vi "perform asynchronous fault handling.vi"(0 "module in":T2, 1 "fault fifo":refnum<k33>, 2 "error classification":T1, 3 "iteration":u64, 5 "module ref in":refnum<data-value>, 7 "code":i32, 9 "fault handling in":T4, 11 "run flags in":u8, 12 "engine error in":errorcluster, 13 "engine reference":i32, 14 "cfg ref":refnum<data-value>) -> (4 "module out":T2, 6 "go to safe state":bool, 8 "code out":i32, 10 "engine error out":errorcluster, 15 "run flags out":u8)   [LabVIEW 2013, in "main engine.lvlib"]
uses:
  main engine/main engine.lvlib
  fault handling spec.ctl
  Configuration/Error Actions.ctl
  rt fault.ctl
  <vilib>/NI/Tag Bus Module Framework/runtime/error classification.ctl
  <vilib>/NI/Tag Bus Module Framework/module configuration/TBM module configuration.lvclass
  <vilib>/NI/Tag Bus Module Framework/runtime/TBM module execution interface.lvclass
  async executor/asynchronous executor reference.ctl
  async executor/message to executor.ctl
  async command notification.ctl
  <vilib>/NI/Tag Bus/table/data table.ctl
  async error info.ctl
  <vilib>/NI/Tag Bus/buffer exchange/buffer reference.ctl
  Configuration/Standard Engine Configuration.lvclass
  <vilib>/NI/Tag Bus/table/data table.lvlib
  <vilib>/NI/Tag Bus/buffer exchange/tag bus buffer exchange.lvlib
  async executor/async executor.lvlib
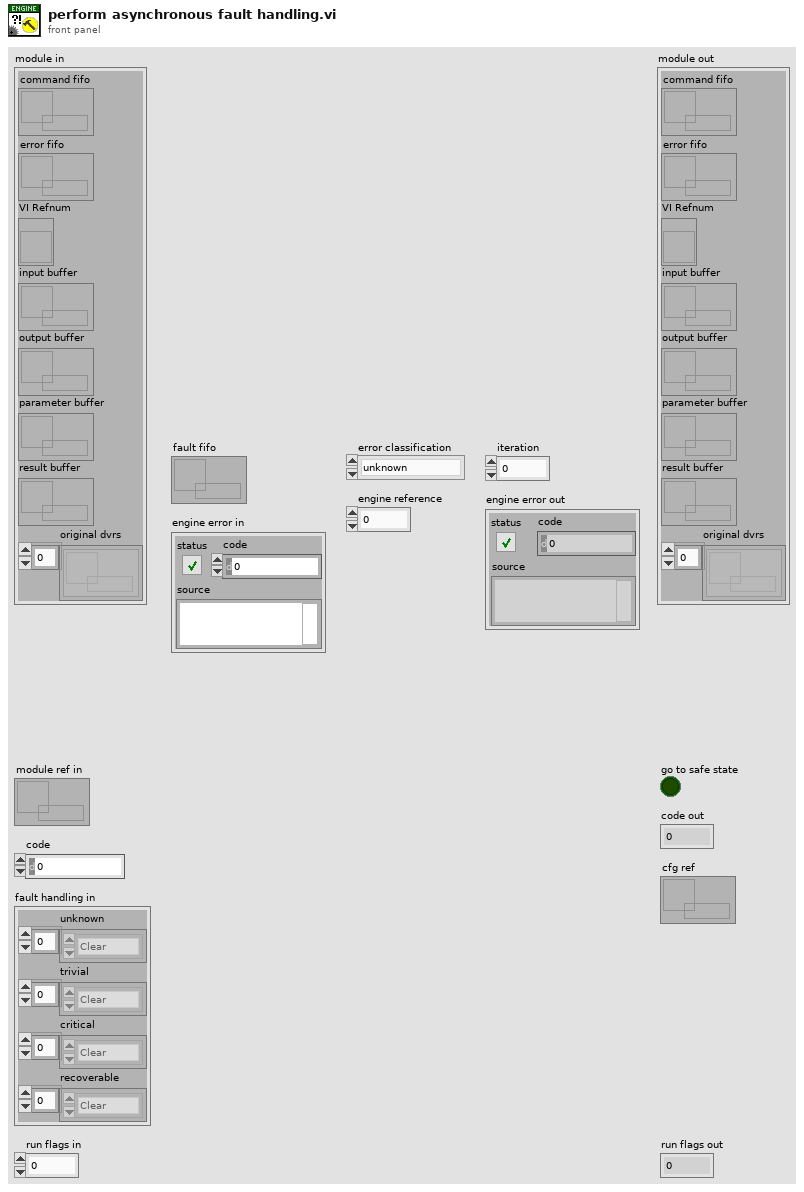
[diagram p1: front panel]
types:
  T1 = typedef "TBM module execution interface.lvclass/error classification.ctl" = enum16{"unknown", "none", "trivial", "recoverable", "critical"}
  T2 = typedef "async executor.lvlib/asynchronous executor reference.ctl" = cluster{"command fifo":refnum<k33>, "error fifo":refnum<k33>, "VI Refnum":refnum<vi>, "input buffer":refnum<k33>, "output buffer":refnum<k33>, "parameter buffer":refnum<k33>, "result buffer":refnum<k33>, "original dvrs":T3[]}
  T3 = typedef "tag bus buffer exchange.lvlib/buffer reference.ctl" = refnum<data-value>
  T4 = typedef "main engine.lvlib/fault handling spec.ctl" = cluster{"unknown":T5[], "trivial":T5[], "critical":T5[], "recoverable":T5[]}
  T5 = typedef "Standard Engine Configuration.lvclass/Error Actions.ctl" = enum16{"Clear", "Notify", "Stop Component", "Stop Engine", "Safe State", "Attempt Recovery"}
  T6 = typedef "main engine.lvlib/rt fault.ctl" = cluster{"code":i32, "classification":T1, "iteration":u64, "cfg ref":refnum<data-value>}
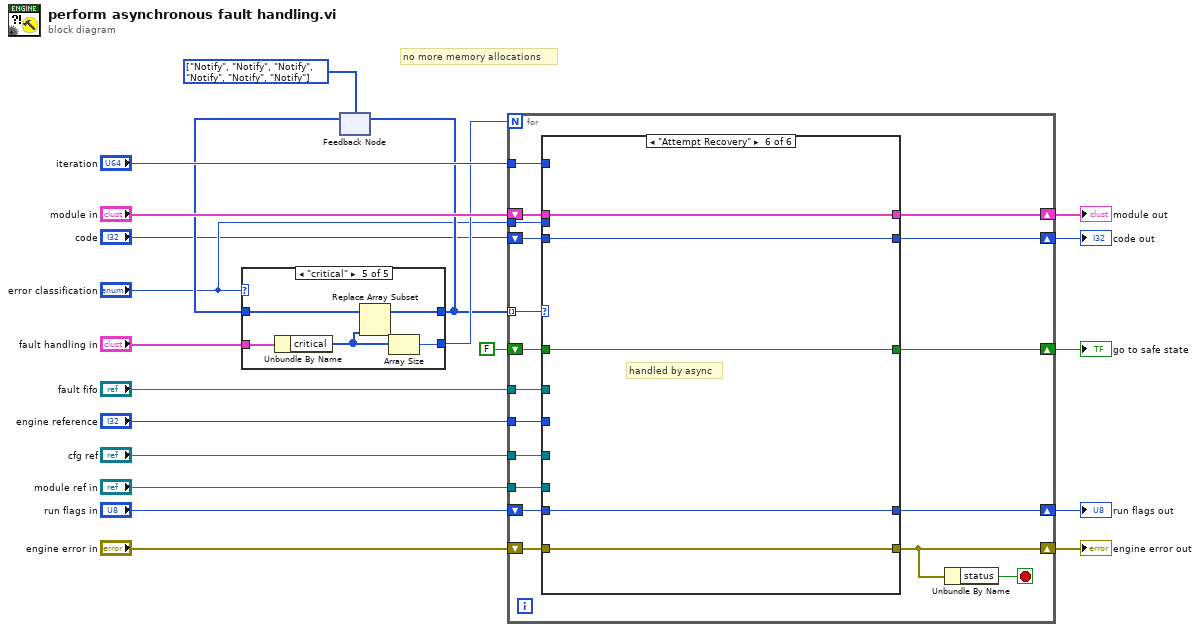
[diagram p0: block diagram]
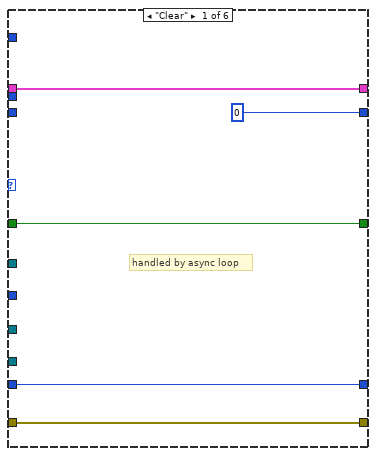
[diagram p2: hidden frame]
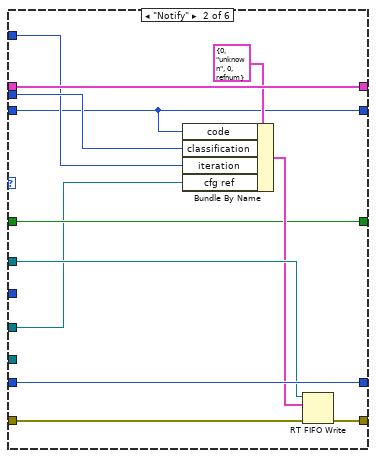
[diagram p3: hidden frame]
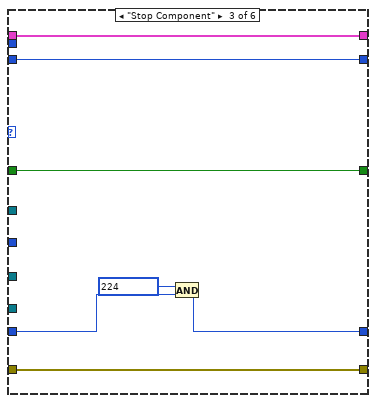
[diagram p4: hidden frame]
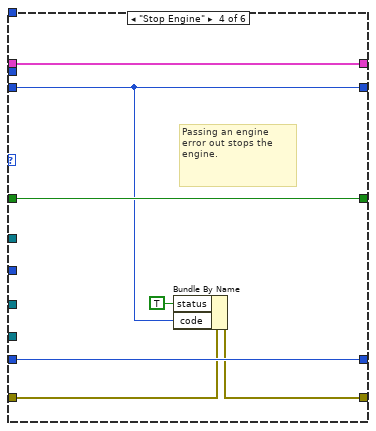
[diagram p5: hidden frame]
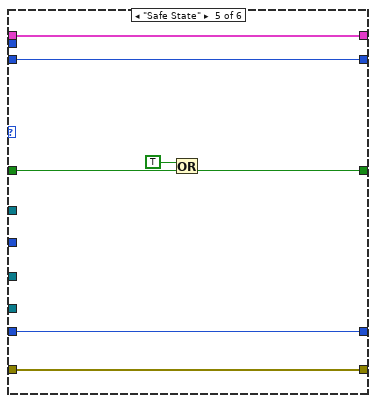
[diagram p6: hidden frame]
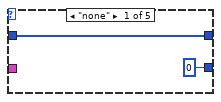
[diagram p7: hidden frame]
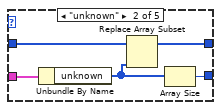
[diagram p8: hidden frame]
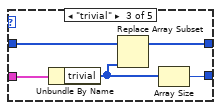
[diagram p9: hidden frame]
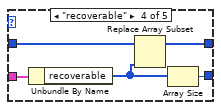
[diagram p10: hidden frame]
diagram:
  w4 = T5[] [enum."Notify", enum."Notify", enum."Notify", enum."Notify", enum."Notify", enum."Notify"] items=["Clear", "Notify", "Stop Component", "Stop Engine", "Safe State", "Attempt Recovery"] ("critical")
  # "no more memory allocations"
  n1 = feedback #1(w4) -> (w5:T5[])
  n2 = case shown="\"critical\"" "error classification" {
    tunnel: "fault handling in" -> [_ w28 w33 w38 w43]
    tunnel: [w22 w25 w30 w35 w40] -> w6
    tunnel: [0 w27 w32 w37 w42] -> w7
    tunnel: w5 -> [w22 w26 w31 w36 w41]
    frame "none" {
    }
    frame "unknown" {
      n3 = Unbundle By Name(w28) -> ("unknown"=w24:T5[])
      n4 = Replace Array Subset(array=w26, new element=w24) -> (w25:T5[])  [unwired: 1 in]
      n5 = Array Size(array=w24) -> (size(s)=w27:i32)
    }
    frame "trivial" {
      n6 = Unbundle By Name(w33) -> ("trivial"=w29:T5[])
      n7 = Replace Array Subset(array=w31, new element=w29) -> (w30:T5[])  [unwired: 1 in]
      n8 = Array Size(array=w29) -> (size(s)=w32:i32)
    }
    frame "recoverable" {
      n9 = Unbundle By Name(w38) -> ("recoverable"=w34:T5[])
      n10 = Replace Array Subset(array=w36, new element=w34) -> (w35:T5[])  [unwired: 1 in]
      n11 = Array Size(array=w34) -> (size(s)=w37:i32)
    }
    frame "critical" {
      n12 = Unbundle By Name(w43) -> ("critical"=w39:T5[])
      n13 = Replace Array Subset(array=w41, new element=w39) -> (w40:T5[])  [unwired: 1 in]
      n14 = Array Size(array=w39) -> (size(s)=w42:i32)
    }
  }
  n15 = feedback-in #1(w6) -> ()
  n16 = for {
    N: w7 -> [_]
    shift-right: [w54] -> w16
    shift-left: "run flags in" -> [w55]
    shift-right: [w57] -> w1
    shift-left: "code" -> [w58]
    shift-right: [w60] -> w17
    shift-left: "module in" -> [w59]
    tunnel: "fault fifo" -> [w51]
    tunnel: w6 -> [w61] mode=indexing
    shift-right: [w52] -> w13
    shift-left: "engine error in" -> [w53]
    tunnel: "error classification" -> [w50]
    tunnel: "iteration" -> [w49]
    shift-right: [w48] -> w10
    shift-left: FALSE -> [w47]
    tunnel: "cfg ref" -> [w46]
    tunnel: "module ref in" -> [w56]
    tunnel: "engine reference" -> [w45]
    stop <- w44 stop-if-true
    n17 = case shown="\"Attempt Recovery\"" w61 {
      tunnel: [w63 w78 w85 w92 w99 w100] -> w60
      tunnel: w59 -> [w63 w78 w85 w92 w99 w100]
      tunnel: w58 -> [_ w67 w84 w86 w98 w104]
      tunnel: [0 ("code") w67 w84 w86 w98 w104] -> w57
      tunnel: w56 -> [_ _ _ _ _ _]
      tunnel: w55 -> [w66 w77 w83 w91 w97 w102]
      tunnel: [w66 w77 w80 w91 w97 w102] -> w54
      tunnel: w53 -> [w65 w76 w82 w88 w96 w101]
      tunnel: [w65 w75 w82 w89 w96 w101] -> w52
      tunnel: w51 -> [_ w74 _ _ _ _]
      tunnel: w50 -> [_ w71 _ _ _ _]
      tunnel: w49 -> [_ w70 _ _ _ _]
      tunnel: [w64 w69 w81 w90 w94 w103] -> w48
      tunnel: w47 -> [w64 w69 w81 w90 w95 w103]
      tunnel: w46 -> [_ w68 _ _ _ _]
      tunnel: w45 -> [_ _ _ _ _ _]
      frame "Clear" {
        # "handled by async loop"
      }
      frame "Notify" {
        n18 = Bundle By Name(cluster=T6 {"code"=0, "classification"=enum."unknown", "iteration"=0, "cfg ref"=refnum} ("element"), "code"=w67, "classification"=w71, "iteration"=w70, "cfg ref"=w68) -> (w72:T6)
        n19 = RT FIFO Write(0:w74, 1:w72, 3:w76) -> (11:w75:errorcluster)  [unwired: 2 in, 3 out]
      }
      frame "Stop Component" {
        n20 = And(x=u8 224, y=w83) -> (x .and. y?=w80:u8)
      }
      frame "Stop Engine" {
        # "Passing an engine error out stops the engine."
        n21 = Bundle By Name(cluster=w88, "status"=TRUE, "code"=w86) -> (w89:errorcluster)
      }
      frame "Safe State" {
        n22 = Or(x=TRUE, y=w95) -> (x .or. y?=w94:bool)
      }
      frame "Attempt Recovery" {
        # "handled by async"
      }
    }
    n23 = Unbundle By Name(w52) -> ("status"=w44:bool)
  }
  "module out" <- w17
  "run flags out" <- w16
  "engine error out" <- w13
  "go to safe state" <- w10
  "code out" <- w1
